vi "UT_Formatter_Main.vi"(8 "error in":errorcluster) -> (0 "error out":errorcluster)   [LabVIEW 2016, in "UT_Formatter.lvlib"]
doc: "Collection of tests for Formatter class."
uses:
  UT_Formatter.lvlib
  <vilib>/addons/_JKI Toolkits/Caraya/classes/Test/Test.lvclass
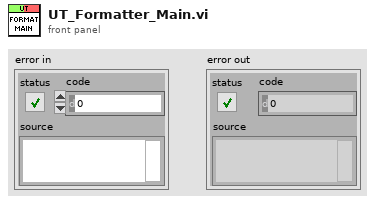
[diagram p1: front panel]
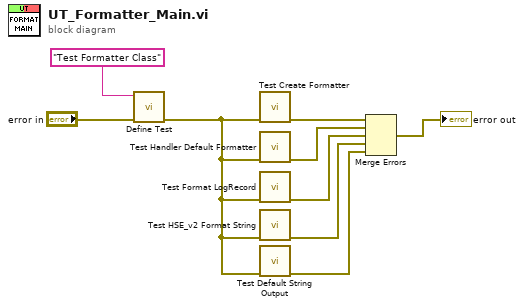
[diagram p0: block diagram]
diagram:
  n1 = call <vilib>:"Define Test.vi"("error in (no error)"="error in", "Label (VI Title)"="Test Formatter Class") -> ("error out"=w2:errorcluster)  [unwired: 8 in, 1 out]
  n2 = call "Test Create Formatter.vi"("error in"=w2) -> ("error out"=w7:errorcluster)  [unwired: 10 in]
  n3 = call "Test Handler Default Formatter.vi"("error in"=w2) -> ("error out"=w5:errorcluster)  [unwired: 10 in]
  n4 = call "Test Format LogRecord.vi"("error in"=w2) -> ("error out"=w6:errorcluster)  [unwired: 10 in]
  n5 = call "Test HSE_v2 Format String.vi"("error in (no error)"=w2) -> ("error out"=w3:errorcluster)  [unwired: 10 in]
  n6 = call "Test Default String Output.vi"("error in (no error)"=w2) -> ("error out"=w1:errorcluster)  [unwired: 10 in]
  n7 = Merge Errors(w7, w5, w6, w3, w1) -> (→"error out":errorcluster)
